vi "Master Setup Open.vi"(11 "Master Setup File (in)":path) -> (2 "File Paths (out)":path[](array[path]), 3 "Master Setup File (out)":path)   [LabVIEW 2017]
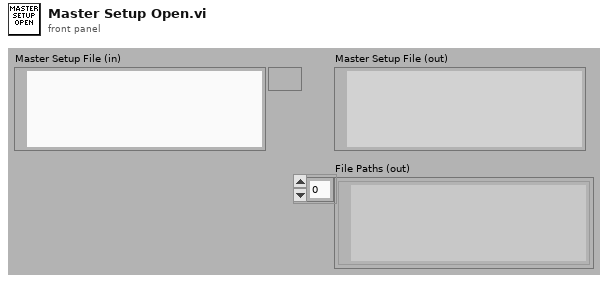
[diagram p1: front panel]
types:
  T1 = enum16{"Load Master Setup", "Check if Files Exist", "Check if File Type is Correct", "Ask to Prompt for Files", "Prompt for Files"}
  T2 = enum16{"open", "replace", "create", "open or create", "replace or create", "replace or create with confirmation"}
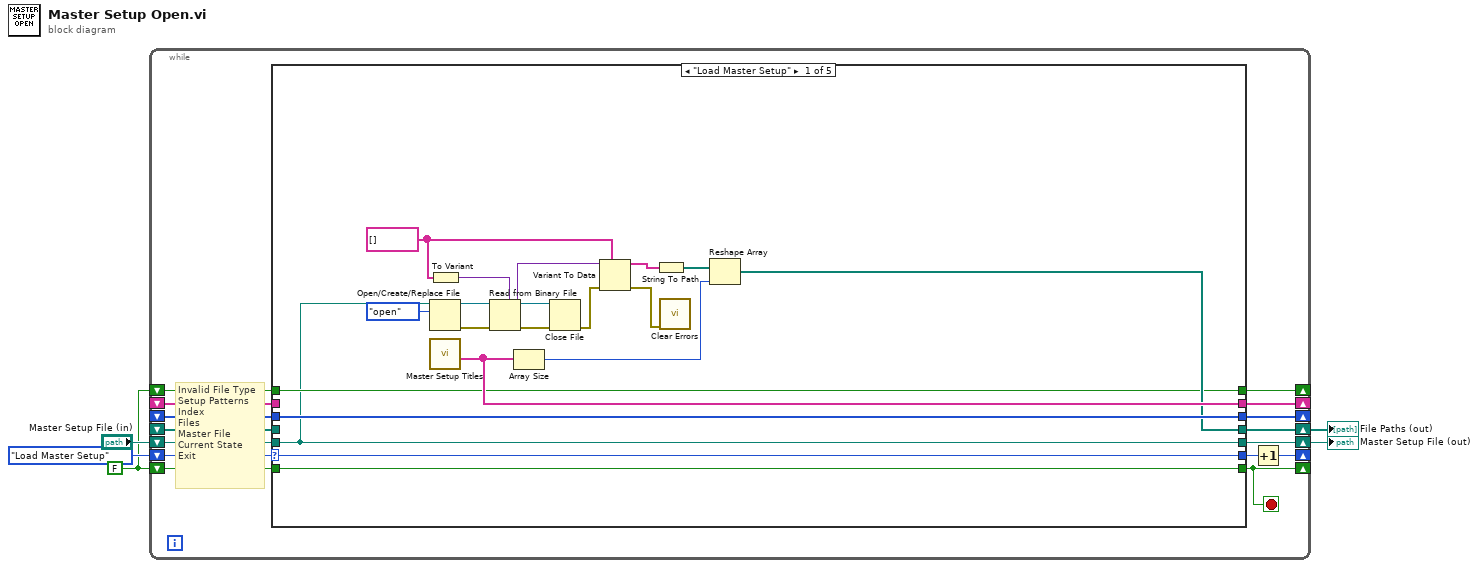
[diagram p0: block diagram]
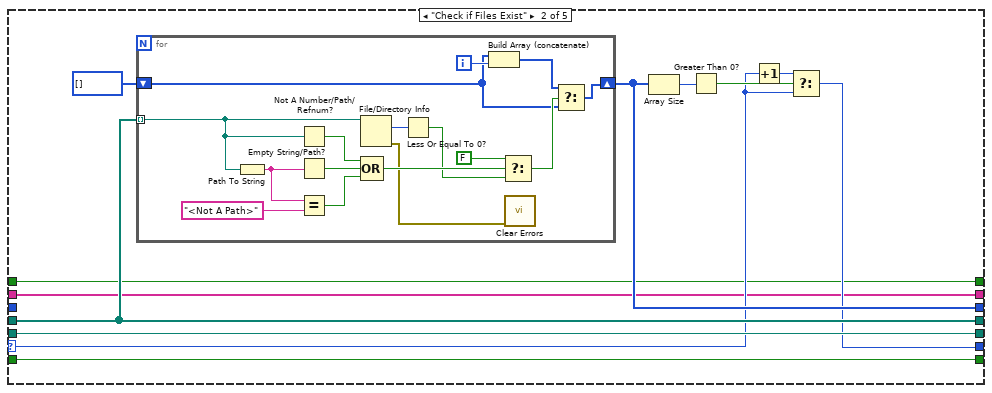
[diagram p2: hidden frame]
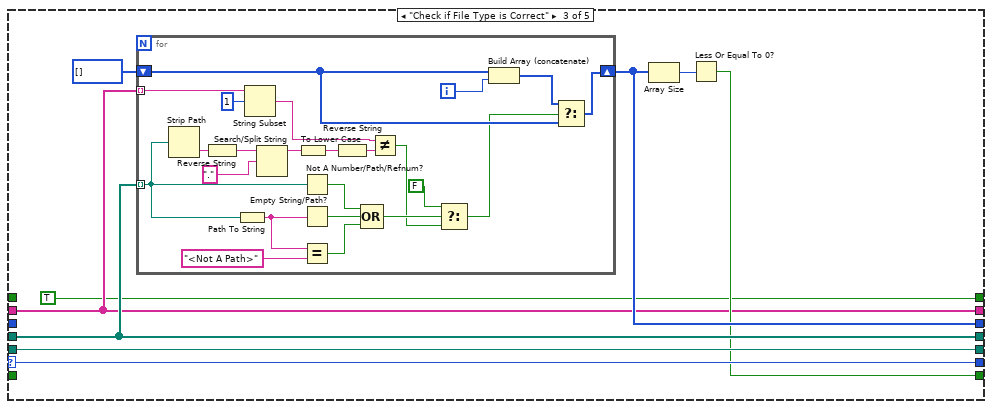
[diagram p3: hidden frame]
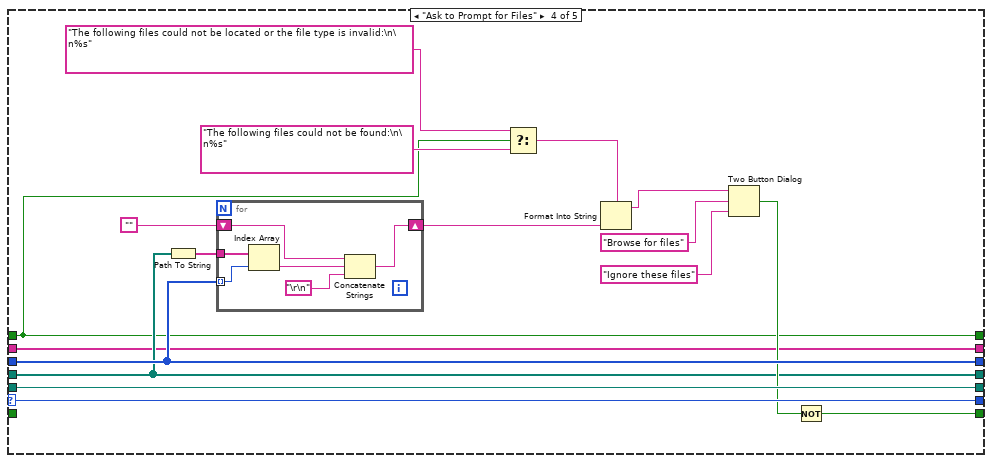
[diagram p4: hidden frame]
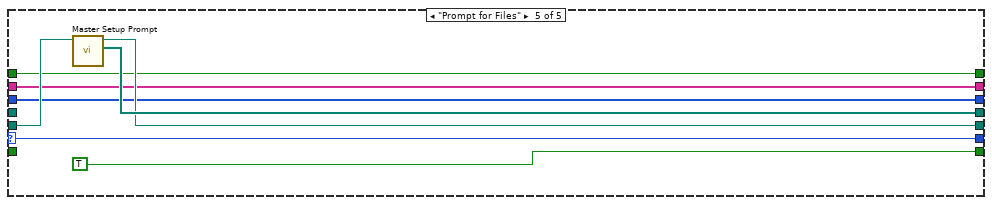
[diagram p5: hidden frame]
diagram:
  w1 = FALSE
  n1 = while {
    shift-right: [w11] -> _
    shift-left: w1 -> [w16]
    shift-right: [w19] -> w2
    shift-left: "Master Setup File (in)" -> [w20]
    shift-right: [w17] -> w3
    shift-left: _ -> [w18]
    shift-right: [w10] -> _
    shift-left: T1."Load Master Setup" -> [w15]
    shift-right: [w12] -> _
    shift-left: _ -> [w14]
    shift-right: [w8] -> _
    shift-left: _ -> [w9]
    shift-right: [w6] -> _
    shift-left: w1 -> [w7]
    stop <- w11 stop-if-true
    # "Invalid File Type\nSetup Patterns\nIndex\nFiles\nMaster File\nCurrent State\nExit"
    n2 = case shown="\"Load Master Setup\"" w15 {
      selector: w15 -> [w39 w44 w72 w116 w128]
      tunnel: w16 -> [w35 w46 _ _ _]
      tunnel: w20 -> [w31 w52 w77 w117 w130]
      tunnel: [w35 w46 w71 w108 TRUE] -> w11
      tunnel: [w31 w52 w77 w117 w129] -> w19
      tunnel: w18 -> [_ w51 w76 w107 _]
      tunnel: [w37 w51 w76 w107 w131] -> w17
      tunnel: w14 -> [w40 _ _ w115 w126]
      tunnel: [w39 w45 w72 w116 w128] -> w13
      tunnel: [w40 w49 w74 w115 w126] -> w12
      tunnel: w9 -> [_ w42 w70 w105 w125]
      tunnel: [w38 w42 w70 w105 w125] -> w8
      tunnel: w7 -> [w36 w41 _ w103 w124]
      tunnel: [w36 w41 TRUE w103 w124] -> w6
      frame "Load Master Setup" {
        w26 = string[] []
        n3 = Open/Create/Replace File(file path (use dialog)=w31, operation (0:open)=T2."open") -> (refnum out=w30:refnum<file>, error out=w34:errorcluster)  [unwired: 4 in, 1 out]
        n4 = call "Master Setup Titles.vi"() -> ("Setup Patterns"=w38:string[])  [unwired: 6 in, 5 out]
        n5 = To Variant(anything=w26) -> (Variant=w28:variant)
        n6 = Read from Binary File(5:w28, 8:w34, 11:w30) -> (0:w33:errorcluster, 2:w27:variant, 3:w32:refnum<file>)  [unwired: 3 in, 1 out]
        n7 = Array Size(array=w38) -> (size(s)=w21:i32)
        n8 = Close File(refnum=w32, error in=w33) -> (error out=w23:errorcluster)  [unwired: 1 out]
        n9 = Variant To Data(error in=w23, type=w26, Variant=w27) -> (data=w25:string[], error out=w22:errorcluster)
        n10 = String To Path(string=w25) -> (path=w24:path[])
        n11 = call <vilib>:"Clear Errors.vi"("error in (no error)"=w22) -> ()  [unwired: 5 in, 2 out]
        n12 = Reshape Array(w24, w21) -> (w37:path[])
      }
      frame "Check if Files Exist" {
        n13 = for {
          tunnel: w51 -> [w63] mode=indexing
          shift-right: [w55] -> w49
          shift-left: i32[] [] -> [w54]
          i -> [w57]
          n14 = Path To String(path=w63) -> (string=w66:string)
          n15 = Not A Number/Path/Refnum?(number/path/refnum=w63) -> (NaN/Path/Refnum?=w67:bool)
          n16 = Empty String/Path?(string/path=w66) -> (empty?=w68:bool)
          n17 = Equal?(x=w66, y="<Not A Path>") -> (x = y?=w64:bool)
          n18 = File/Directory Info(path=w63) -> (size=w62:i64, error out=w53:errorcluster)  [unwired: 1 in, 5 out]
          n19 = Compound Arithmetic op=OR(w67, w68, w64) -> (w61:bool)
          n20 = Less Or Equal To 0?(x=w62) -> (x <= 0?=w60:bool)
          n21 = Build Array (concatenate)(w54, w57) -> (w56:i32[])
          n22 = Select(t=FALSE, s=w61, f=w60) -> (s? t:f=w58:bool)
          n23 = call <vilib>:"Clear Errors.vi"("error in (no error)"=w53) -> ()  [unwired: 5 in, 2 out]
          n24 = Select(t=w56, s=w58, f=w54) -> (s? t:f=w55:i32[])
        }
        n25 = Array Size(array=w49) -> (size(s)=w48:i32)
        n26 = Greater Than 0?(x=w48) -> (x > 0?=w47:bool)
        n27 = Increment(x=w44) -> (x+1=w43:T1)
        n28 = Select(t=w43, s=w47, f=w44) -> (s? t:f=w45:T1)
      }
      frame "Check if File Type is Correct" {
        n29 = for {
          tunnel: w76 -> [w91] mode=indexing
          shift-right: [w93] -> w74
          shift-left: i32[] [] -> [w92]
          tunnel: w70 -> [w80] mode=indexing
          i -> [w95]
          n30 = Strip Path(path=w91) -> (name=w83:string)  [unwired: 1 out]
          n31 = Reverse String(1:w83) -> (0:w84:string)
          n32 = Path To String(path=w91) -> (string=w98:string)
          n33 = String Subset(string=w80, offset (0)=1) -> (substring=w79:string)  [unwired: 1 in]
          n34 = Search/Split String(string=w84, search string/char (-)=".") -> (substring before match=w81:string)  [unwired: 1 in, 2 out]
          n35 = To Lower Case(string=w81) -> (all lower case string=w90:string)
          n36 = Not A Number/Path/Refnum?(number/path/refnum=w91) -> (NaN/Path/Refnum?=w99:bool)
          n37 = Empty String/Path?(string/path=w98) -> (empty?=w100:bool)
          n38 = Equal?(x=w98, y="<Not A Path>") -> (x = y?=w96:bool)
          n39 = Reverse String(1:w90) -> (0:w82:string)
          n40 = Compound Arithmetic op=OR(w99, w100, w96) -> (w89:bool)
          n41 = Not Equal?(x=w79, y=w82) -> (x != y?=w88:bool)
          n42 = Select(t=FALSE, s=w89, f=w88) -> (s? t:f=w86:bool)
          n43 = Build Array (concatenate)(w92, w95) -> (w94:i32[])
          n44 = Select(t=w94, s=w86, f=w92) -> (s? t:f=w93:i32[])
        }
        n45 = Array Size(array=w74) -> (size(s)=w73:i32)
        n46 = Less Or Equal To 0?(x=w73) -> (x <= 0?=w71:bool)
      }
      frame "Ask to Prompt for Files" {
        n47 = Path To String(path=w107) -> (string=w106:string[])
        n48 = for {
          tunnel: w115 -> [w122] mode=indexing
          tunnel: w106 -> [w123]
          shift-right: [w119] -> w113
          shift-left: "" -> [w118]
          n49 = Index Array(array=w123, index=w122) -> (element=w121:string)
          n50 = Concatenate Strings(w118, w121, "\r\n") -> (w119:string)
        }
        n51 = Select(t="The following files could not be located or the file type is invalid:\n\n%s" ("format string"), s=w103, f="The following files could not be found:\n\n%s" ("format string")) -> (s? t:f=w101:string)
        n52 = Format Into String(format string=w101, w113) -> (resulting string=w112:string)  [unwired: 2 in, 1 out]
        n53 = Two Button Dialog(message=w112, 1:"Ignore these files" ("T button name (\"OK\")"), 2:"Browse for files" ("T button name (\"OK\")")) -> (T button?=w109:bool)
        n54 = Not(x=w109) -> (.not. x?=w108:bool)
      }
      frame "Prompt for Files" {
        n55 = call "Master Setup Prompt.vi"("Master Setup File (in)"=w130) -> ("Current File Paths"=w131:path[], "Master Setup File (out)"=w129:path)  [unwired: 5 in]
      }
    }
    n56 = Increment(x=w13) -> (x+1=w10:T1)
  }
  "File Paths (out)" <- w3
  "Master Setup File (out)" <- w2
